vi "Binary Clock.vi"() -> ()   [LabVIEW 2010]
panel:
  in  "stop":bool
  in  "Lap":bool
  out "Array 7":bool[](array[boolean])
  out "Array 6":bool[](array[boolean])
  out "Array 4":bool[](array[boolean])
  out "Array 3":bool[](array[boolean])
  out "Array 2":bool[](array[boolean])
  out "Array":bool[](array[boolean])
  # "8"
  # "4"
  # "2"
  # "1"
  # "Hours"
  # "Minutes"
  # "Seconds"
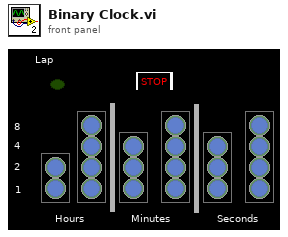
[diagram p1: front panel]
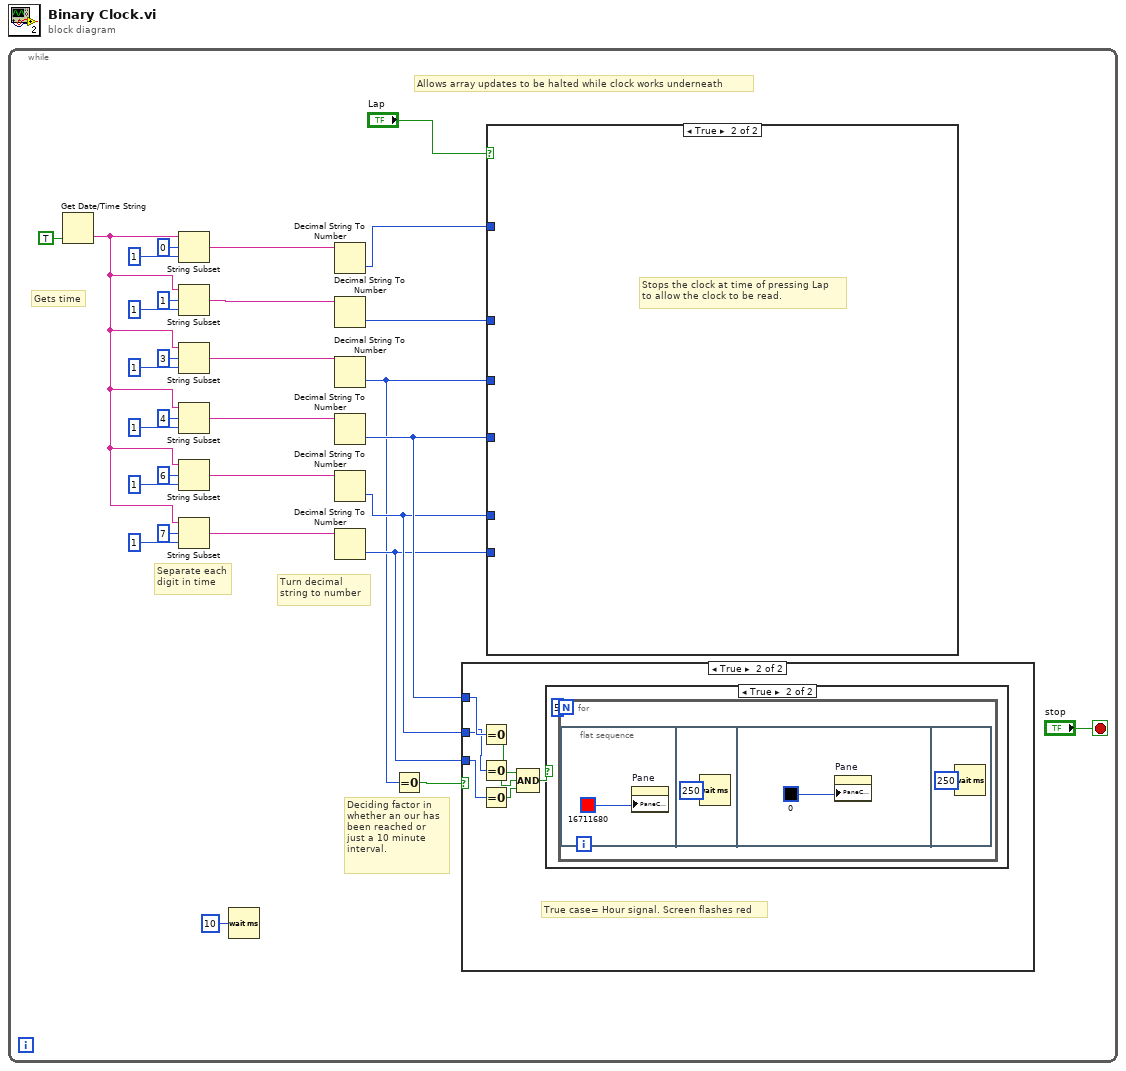
[diagram p0: block diagram]
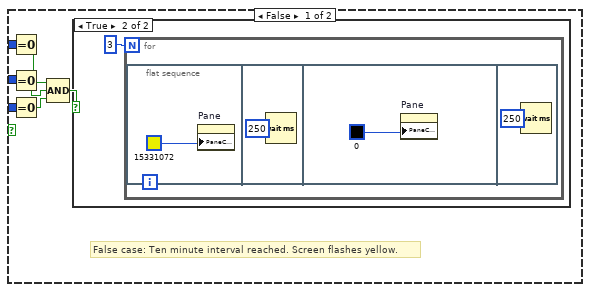
[diagram p2: hidden frame]
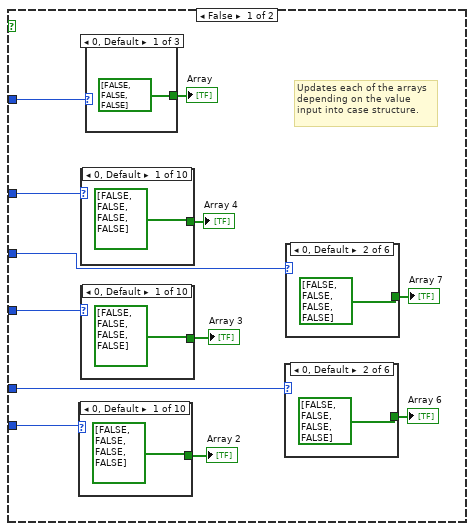
[diagram p5: hidden frame]
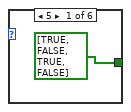
[diagram p6: hidden frame]
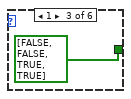
[diagram p7: hidden frame]
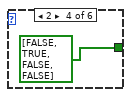
[diagram p8: hidden frame]
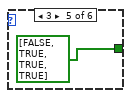
[diagram p9: hidden frame]
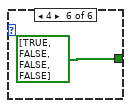
[diagram p10: hidden frame]
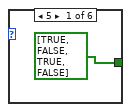
[diagram p11: hidden frame]
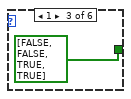
[diagram p12: hidden frame]
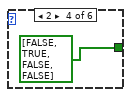
[diagram p13: hidden frame]
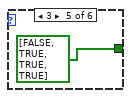
[diagram p14: hidden frame]
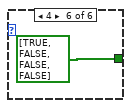
[diagram p15: hidden frame]
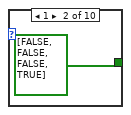
[diagram p16: hidden frame]
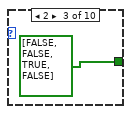
[diagram p17: hidden frame]
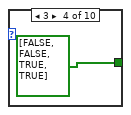
[diagram p18: hidden frame]
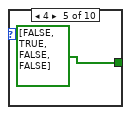
[diagram p19: hidden frame]
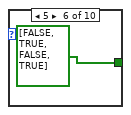
[diagram p20: hidden frame]
diagram:
  n1 = while {
    stop <- "stop" stop-if-true
    # "Deciding factor in\nwhether an our has\nbeen reached or\njust a 10 minute \ninterval."
    # "Allows array updates to be halted while clock works underneath"
    # "Turn decimal \nstring to number"
    # "Separate each\ndigit in time"
    # "Gets time"
    n2 = Get Date/Time String(want seconds? (F)=TRUE) -> (time string=w17:string)  [unwired: 2 in, 1 out]
    n3 = String Subset(string=w17, offset (0)=0, length (rest)=1 ("length (rest)")) -> (substring=w16:string)
    n4 = String Subset(string=w17, offset (0)=1, length (rest)=1 ("length (rest)")) -> (substring=w15:string)
    n5 = String Subset(string=w17, offset (0)=3, length (rest)=1 ("length (rest)")) -> (substring=w14:string)
    n6 = String Subset(string=w17, offset (0)=4, length (rest)=1 ("length (rest)")) -> (substring=w13:string)
    n7 = String Subset(string=w17, offset (0)=6, length (rest)=1 ("length (rest)")) -> (substring=w12:string)
    n8 = String Subset(string=w17, offset (0)=7, length (rest)=1 ("length (rest)")) -> (substring=w11:string)
    n9 = Wait (ms)(milliseconds to wait=u32 10) -> ()  [unwired: 1 out]
    n10 = Decimal String To Number(string=w16) -> (number=w10:i32)  [unwired: 2 in, 1 out]
    n11 = Decimal String To Number(string=w15) -> (number=w9:i32)  [unwired: 2 in, 1 out]
    n12 = Decimal String To Number(string=w14) -> (number=w3:i32)  [unwired: 2 in, 1 out]
    n13 = Decimal String To Number(string=w13) -> (number=w6:i32)  [unwired: 2 in, 1 out]
    n14 = Decimal String To Number(string=w12) -> (number=w5:i32)  [unwired: 2 in, 1 out]
    n15 = Decimal String To Number(string=w11) -> (number=w4:i32)  [unwired: 2 in, 1 out]
    n16 = Equal To 0?(x=w3) -> (x = 0?=w2:bool)
    n17 = case shown="True" w2 {
      tunnel: w6 -> [w37 w46]
      tunnel: w5 -> [w36 w45]
      tunnel: w4 -> [w35 w44]
      frame False {
        # "False case: Ten minute interval reached. Screen flashes yellow."
        n18 = Equal To 0?(x=w37) -> (x = 0?=w34:bool)
        n19 = Equal To 0?(x=w36) -> (x = 0?=w33:bool)
        n20 = Equal To 0?(x=w35) -> (x = 0?=w32:bool)
        n21 = Compound Arithmetic op=AND(w34, w33, w32) -> (w31:bool)
        n22 = case shown="True" w31 {
          frame False {
            # "Continues to run with black background"
          }
          frame True {
            n23 = for {
              N: 3 ("Numeric") -> [_]
              n24 = flat-sequence {
                frame #0 {
                  n25 = property on="Pane" class="Pane"("PaneColor"=u32 15331072) -> ()  [unwired: 2 in, 2 out]
                }
                frame #1 {
                  n26 = Wait (ms)(milliseconds to wait=u32 250) -> ()  [unwired: 1 out]
                }
                frame #2 {
                  n27 = property on="Pane" class="Pane"("PaneColor"=u32 0) -> ()  [unwired: 2 in, 2 out]
                }
                frame #3 {
                  n28 = Wait (ms)(milliseconds to wait=u32 250) -> ()  [unwired: 1 out]
                }
              }
            }
          }
        }
      }
      frame True {
        # "True case= Hour signal. Screen flashes red"
        n29 = Equal To 0?(x=w46) -> (x = 0?=w49:bool)
        n30 = Equal To 0?(x=w45) -> (x = 0?=w48:bool)
        n31 = Equal To 0?(x=w44) -> (x = 0?=w47:bool)
        n32 = Compound Arithmetic op=AND(w49, w48, w47) -> (w43:bool)
        n33 = case shown="True" w43 {
          frame False {
            # "Continues to run with black background"
          }
          frame True {
            n34 = for {
              N: 5 -> [_]
              n35 = flat-sequence {
                frame #0 {
                  n36 = property on="Pane" class="Pane"("PaneColor"=u32 16711680) -> ()  [unwired: 2 in, 2 out]
                }
                frame #1 {
                  n37 = Wait (ms)(milliseconds to wait=u32 250) -> ()  [unwired: 1 out]
                }
                frame #2 {
                  n38 = property on="Pane" class="Pane"("PaneColor"=u32 0) -> ()  [unwired: 2 in, 2 out]
                }
                frame #3 {
                  n39 = Wait (ms)(milliseconds to wait=u32 250) -> ()  [unwired: 1 out]
                }
              }
            }
          }
        }
      }
    }
    n40 = case shown="True" "Lap" {
      tunnel: w10 -> [w66 _]
      tunnel: w4 -> [w65 _]
      tunnel: w6 -> [w61 _]
      tunnel: w9 -> [w60 _]
      tunnel: w5 -> [w57 _]
      tunnel: w3 -> [w55 _]
      frame False {
        # "Updates each of the arrays\ndepending on the value\ninput into case structure."
        n41 = case shown="0, Default" w65 {
          tunnel: [bool[] [FALSE, FALSE, FALSE, FALSE] ("Array") bool[] [FALSE, FALSE, FALSE, TRUE] ("Array") bool[] [FALSE, FALSE, TRUE, FALSE] ("Array") bool[] [FALSE, FALSE, TRUE, TRUE] ("Array") bool[] [FALSE, TRUE, FALSE, FALSE] ("Array") bool[] [FALSE, TRUE, FALSE, TRUE] ("Array") bool[] [FALSE, TRUE, TRUE, FALSE] ("Array") bool[] [FALSE, TRUE, TRUE, TRUE] ("Array") bool[] [TRUE, FALSE, FALSE, FALSE] ("Array") bool[] [TRUE, FALSE, FALSE, TRUE] ("Array")] -> w63
          frame 0, Default {
          }
          frame 1 {
          }
          frame 2 {
          }
          frame 3 {
          }
          frame 4 {
          }
          frame 5 {
          }
          frame 6 {
          }
          frame 7 {
          }
          frame 8 {
          }
          frame 9 {
          }
        }
        "Array 2" <- w63
        n42 = case shown="0, Default" w60 {
          tunnel: [bool[] [FALSE, FALSE, FALSE, FALSE] ("Array") bool[] [FALSE, FALSE, FALSE, TRUE] ("Array") bool[] [FALSE, FALSE, TRUE, FALSE] ("Array") bool[] [FALSE, FALSE, TRUE, TRUE] ("Array") bool[] [FALSE, TRUE, FALSE, FALSE] ("Array") bool[] [FALSE, TRUE, FALSE, TRUE] ("Array") bool[] [FALSE, TRUE, TRUE, FALSE] ("Array") bool[] [FALSE, TRUE, TRUE, TRUE] ("Array") bool[] [TRUE, FALSE, FALSE, FALSE] ("Array") bool[] [TRUE, FALSE, FALSE, TRUE] ("Array")] -> w59
          frame 0, Default {
          }
          frame 1 {
          }
          frame 2 {
          }
          frame 3 {
          }
          frame 4 {
          }
          frame 5 {
          }
          frame 6 {
          }
          frame 7 {
          }
          frame 8 {
          }
          frame 9 {
          }
        }
        "Array 4" <- w59
        n43 = case shown="0, Default" w61 {
          tunnel: [bool[] [FALSE, FALSE, FALSE, FALSE] ("Array") bool[] [FALSE, FALSE, FALSE, TRUE] ("Array") bool[] [FALSE, FALSE, TRUE, FALSE] ("Array") bool[] [FALSE, FALSE, TRUE, TRUE] ("Array") bool[] [FALSE, TRUE, FALSE, FALSE] ("Array") bool[] [FALSE, TRUE, FALSE, TRUE] ("Array") bool[] [FALSE, TRUE, TRUE, FALSE] ("Array") bool[] [FALSE, TRUE, TRUE, TRUE] ("Array") bool[] [TRUE, FALSE, FALSE, FALSE] ("Array") bool[] [TRUE, FALSE, FALSE, TRUE] ("Array")] -> w62
          frame 0, Default {
          }
          frame 1 {
          }
          frame 2 {
          }
          frame 3 {
          }
          frame 4 {
          }
          frame 5 {
          }
          frame 6 {
          }
          frame 7 {
          }
          frame 8 {
          }
          frame 9 {
          }
        }
        "Array 3" <- w62
        n44 = case shown="0, Default" w66 {
          tunnel: [bool[] [FALSE, FALSE, FALSE] ("Array") bool[] [FALSE, TRUE, TRUE] ("Array") bool[] [TRUE, FALSE, FALSE] ("Array")] -> w64
          frame 0, Default {
          }
          frame 1 {
          }
          frame 2 {
          }
        }
        "Array" <- w64
        n45 = case shown="0, Default" w57 {
          tunnel: [bool[] [TRUE, FALSE, TRUE, FALSE] ("Array") bool[] [FALSE, FALSE, FALSE, FALSE] ("Array") bool[] [FALSE, FALSE, TRUE, TRUE] ("Array") bool[] [FALSE, TRUE, FALSE, FALSE] ("Array") bool[] [FALSE, TRUE, TRUE, TRUE] ("Array") bool[] [TRUE, FALSE, FALSE, FALSE] ("Array")] -> w58
          frame 5 {
          }
          frame 0, Default {
          }
          frame 1 {
          }
          frame 2 {
          }
          frame 3 {
          }
          frame 4 {
          }
        }
        "Array 6" <- w58
        n46 = case shown="0, Default" w55 {
          tunnel: [bool[] [TRUE, FALSE, TRUE, FALSE] ("Array") bool[] [FALSE, FALSE, FALSE, FALSE] ("Array") bool[] [FALSE, FALSE, TRUE, TRUE] ("Array") bool[] [FALSE, TRUE, FALSE, FALSE] ("Array") bool[] [FALSE, TRUE, TRUE, TRUE] ("Array") bool[] [TRUE, FALSE, FALSE, FALSE] ("Array")] -> w56
          frame 5 {
          }
          frame 0, Default {
          }
          frame 1 {
          }
          frame 2 {
          }
          frame 3 {
          }
          frame 4 {
          }
        }
        "Array 7" <- w56
      }
      frame True {
        # "Stops the clock at time of pressing Lap\nto allow the clock to be read."
      }
    }
  }
